vi "TestGUI.vi"(11 "output cluster":T1={"XNET"={"Database"="", "Cluster"="", "Port"="", "Baud rate [Bd]"=0, "Termination"=0, "Incoming Rate"=0, "Outcoming Rate"=0, "Write Decimation"=1}, "Incoming Decimation"=0, "Outgoing Decimation"=0, "Bitfile"={"RT Path"=path "", "RIO Device"=0, "Enable"=FALSE}, "Nodes"={"MonitorTool"={"Network"={"Address"=0, "Name"=0}, "Data"={"IncomingSignals"=[], "IncomingDataRefs"=[], "IncomingDataValues"=[], "OutgoingDataRefs"=[], "OutgoingDataValues"=[], "IncomingFrames"=[], "OutgoingFrames"=[]}, "Command Refs"={"Response Refs"={"Block Data Refs"=[], "Values Array"=[], "# of Channels"=0, "Name"=""}, "Command Refs"={"Block Data Refs"=[], "Values Array"=[], "# of Channels"=0, "Name"=""}, "Command Names"=[], "Response Names"=[]}}, "SimNodes"=[]}} {"Nodes"."MonitorTool"."Command Refs"."Response Refs"."Block Data Refs" format="%.0x"; "Nodes"."MonitorTool"."Data"."IncomingDataRefs"."Data Reference" format="%.0x"; "Nodes"."MonitorTool"."Data"."OutgoingDataRefs"."Data Reference" format="%.0x"; "Nodes"."MonitorTool"."Network"."Name" format="%.0x"; "Nodes"."SimNodes"."Network"."Name" format="%.0x"; "XNET"."Termination" items=["Off", "On"]}) -> ()   [LabVIEW 2013, in "J1939 Addon System Explorer.lvlib"]
uses:
  Shared/Types/Compile Addon Settings.ctl
  Shared/Types/XNET Settings.ctl
  Shared/Types/SysDef FPGA Settings.ctl
  Shared/Types/Compiled.Node Settings.ctl
  Shared/Types/Compiled Monitor Tool Settings.ctl
  Shared/Types/Monitor Settings.ctl
  Shared/Types/Device Settings.ctl
  <vilib>/NI Veristand/Custom Device API/Block Data Reference.ctl
  <vilib>/NI Veristand/Custom Device API/Data Reference.ctl
  Shared/Types/Frame Settings.ctl
  Shared/Types/SysDef Command Settings.ctl
  Shared/Types/Complied Simulated Device Settings.ctl
  Shared/Types/Compiled Simulated Settings.ctl
  J1939 Addon System Explorer.lvlib
  Shared/J1939 Addon Shared.lvlib
  <vilib>/NI Veristand/Custom Device API/Custom Device API.lvlib
panel:
  in  "OK Button":bool
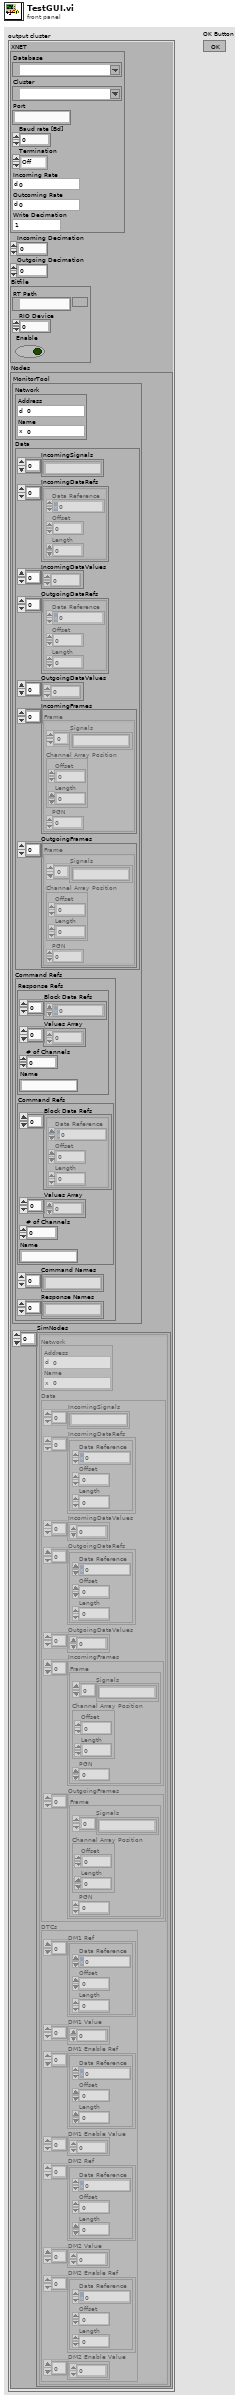
[diagram p1: front panel]
types:
  T1 = typedef "J1939 Addon Shared.lvlib/Compile Addon Settings.ctl" = cluster{"XNET":T2, "Incoming Decimation":u32, "Outgoing Decimation":u32, "Bitfile":T3, "Nodes":T4}
  T2 = typedef "J1939 Addon Shared.lvlib/XNET Settings.ctl" = cluster{"Database":refnum<k21>, "Cluster":refnum<k21>, "Port":string, "Baud rate [Bd]":u32, "Termination":u32, "Incoming Rate":u32, "Outcoming Rate":u32, "Write Decimation":u32}
  T3 = typedef "J1939 Addon Shared.lvlib/SysDef FPGA Settings.ctl" = cluster{"RT Path":path, "RIO Device":u16, "Enable":bool}
  T4 = typedef "J1939 Addon Shared.lvlib/Compiled.Node Settings.ctl" = cluster{"MonitorTool":T5, "SimNodes":T12[]}
  T5 = typedef "J1939 Addon Shared.lvlib/Compiled Monitor Tool Settings.ctl" = cluster{"Network":T6, "Data":T7, "Command Refs":T11}
  T6 = typedef "J1939 Addon Shared.lvlib/Monitor Settings.ctl" = cluster{"Address":u8, "Name":u64}
  T7 = typedef "J1939 Addon Shared.lvlib/Device Settings.ctl" = cluster{"IncomingSignals":string[], "IncomingDataRefs":T8[], "IncomingDataValues":dbl[], "OutgoingDataRefs":T8[], "OutgoingDataValues":dbl[], "IncomingFrames":T10[], "OutgoingFrames":T10[]}
  T8 = typedef "Custom Device API.lvlib/Block Data Reference.ctl" = cluster{"Data Reference":T9, "Offset":i32, "Length":i32}
  T9 = typedef "Custom Device API.lvlib/Data Reference.ctl" = i32
  T10 = typedef "J1939 Addon Shared.lvlib/Frame Settings.ctl" = cluster{"Signals":string[], "Channel Array Position":cluster{"Offset":i32, "Length":i32}, "PGN":u32}
  T11 = typedef "J1939 Addon Shared.lvlib/SysDef Command Settings.ctl" = cluster{"Response Refs":cluster{"Block Data Refs":T9[], "Values Array":dbl[], "# of Channels":u32, "Name":string}, "Command Refs":cluster{"Block Data Refs":T8[], "Values Array":dbl[], "# of Channels":u32, "Name":string}, "Command Names":string[], "Response Names":string[]}
  T12 = typedef "J1939 Addon Shared.lvlib/Complied Simulated Device Settings.ctl" = cluster{"Network":T6, "Data":T7, "DTCs":T13}
  T13 = typedef "J1939 Addon Shared.lvlib/Compiled Simulated Settings.ctl" = cluster{"DM1 Ref":T8[], "DM1 Value":dbl[], "DM1 Enable Ref":T8[], "DM1 Enable Value":dbl[], "DM2 Ref":T8[], "DM2 Value":dbl[], "DM2 Enable Ref":T8[], "DM2 Enable Value":dbl[]}
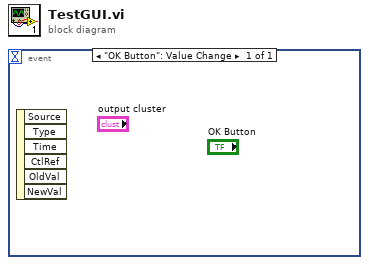
[diagram p0: block diagram]
diagram:
  n1 = event shown="[0] \"OK Button\": Value Change" {
    selector: _ -> [_]
    dyn-events: _ -> [_]
    timeout: _ -> [_]
    event "OK Button": Value Change {
      n2 = event-data() -> ()  [unwired: 1 in, 6 out]
    }
  }
